vi "DSA Clear AI and AO.vi"(0 "AI Task ID In":refnum<k21>[](array[refnum]), 1 "AO Task ID In":refnum<k21>[](array[refnum]), 5 "Errors In":errorcluster[](array[cluster])) -> (19 "Errors Out":errorcluster[](array[cluster]))   [LabVIEW 2014]
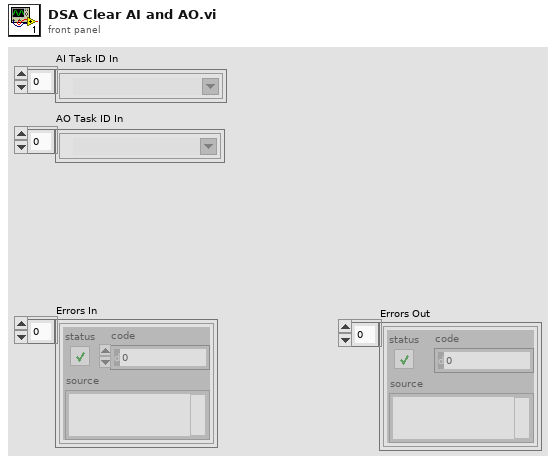
[diagram p1: front panel]
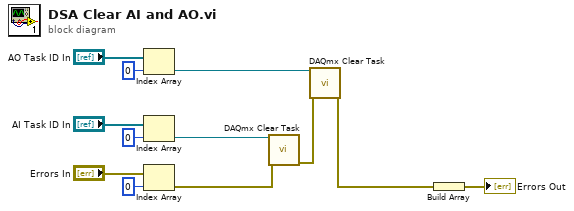
[diagram p0: block diagram]
diagram:
  n1 = Index Array(array="AO Task ID In", index=0) -> (element=w8:refnum<k21>)
  n2 = Index Array(array="AI Task ID In", index=0) -> (element=w7:refnum<k21>)
  n3 = Index Array(array="Errors In", index=0) -> (element=w4:errorcluster)
  n4 = call <vilib>:"DAQmx Clear Task.vi"("task in"=w7, "error in"=w4) -> ("error out"=w1:errorcluster)  [unwired: 13 in]
  n5 = call <vilib>:"DAQmx Clear Task.vi"("task in"=w8, "error in"=w1) -> ("error out"=w3:errorcluster)  [unwired: 13 in]
  n6 = Build Array(w3) -> (→"Errors Out":errorcluster[])
